vi "Write Full Computation.vi"(8 "error in (no error)":errorcluster, 10 "Full Computation?":bool, 11 "Video Cam Processor in":refnum<class "Video Cam Processor.lvclass">) -> (0 "error out":errorcluster, 3 "Video Cam Processor out":refnum<class "Video Cam Processor.lvclass">)   [LabVIEW 2018, in "Video Cam Processor.lvclass"]
uses:
  Video Cam Processor.lvclass
  Video Cam Processor.lvclass/Video Cam Processor.ctl
  Roughness Averager/Roughness Averager.lvclass
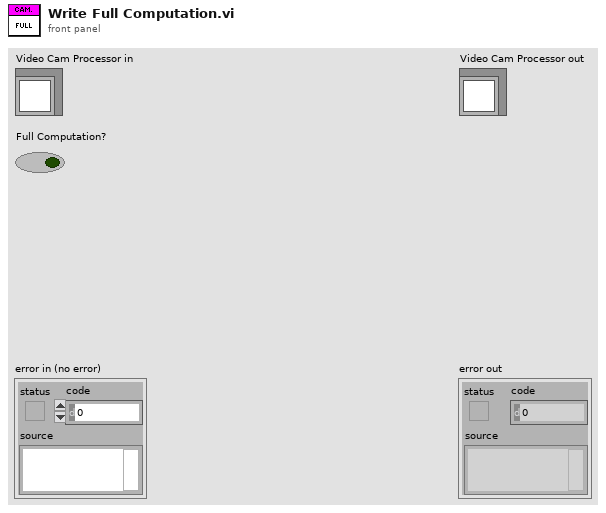
[diagram p1: front panel]
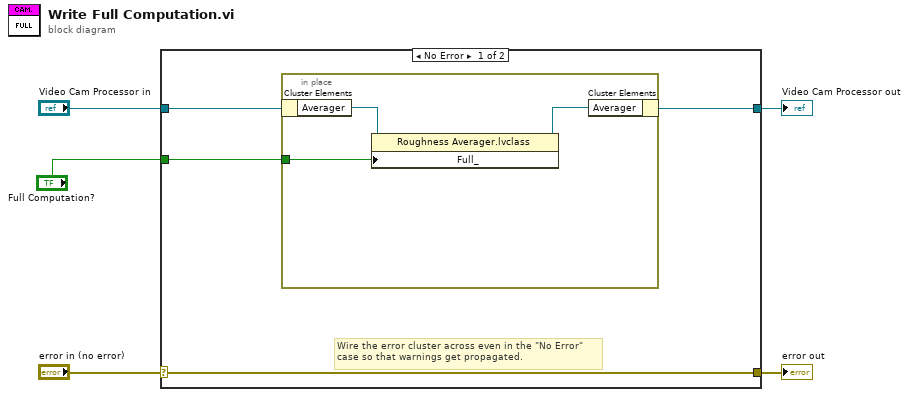
[diagram p0: block diagram]
diagram:
  n1 = case shown="No Error" "error in (no error)" {
    selector: "error in (no error)" -> [w9 w14]
    tunnel: [w9 w14] -> w4
    tunnel: [w7 w13] -> w2
    tunnel: "Video Cam Processor in" -> [w8 w13]
    tunnel: "Full Computation?" -> [w6 _]
    frame No Error {
      # "Wire the error cluster across even in the \"No Error\"\ncase so that warnings get propagated."
      n2 = in-place {
        in-place-border: w6 -> [w10]
        n3 = in-place-cluster #1(w8) -> ("Averager"=w12:refnum<class "Roughness Averager.lvclass">)
        n4 = property class="Roughness Averager.lvclass"(reference=w12, "Full_"=w10) -> (reference out=w11:refnum<class "Roughness Averager.lvclass">)  [unwired: 1 in, 1 out]
        n5 = in-place-cluster #1("Averager"=w11) -> (w7:refnum<class "Video Cam Processor.lvclass">)
      }
    }
    frame Error {
    }
  }
  "error out" <- w4
  "Video Cam Processor out" <- w2
